vi "Initialize.vi"(7 "writer buffer size":i32=4096, 8 "error in (no error)":errorcluster, 10 "reader url":string, 11 "writer name":string) -> (0 "error out":errorcluster, 3 "NetworkStreamWriter out":refnum<class "NetworkStreamWriter.lvclass">)   [LabVIEW 2011, in "NetworkStreamWriter.lvclass"]
doc: "Instantiates an instance of the NetworkStreamWriter class. A NetworkStreamWriter Object is a wrapper around the LabVIEW Network Stream Writer. The wrapper provides a reconnectable connection and separates writes to the Object from network communication. As with network streams, the writer url on the reader or the reader url on the writer must be given in order to establish the connection. The Object will write data across the network stream at a fixed rate in the background. This allows an application to write data to the Object in time-critical loops, as network communication occurs in a separate loop in the background.\n\n<b>It is critical that all initialized NetworkStreamWriter Objects are closed with the Close method.</b> This method signals the background process to stop. If the Close method is not called, the background process will continue to run on the host computer. For this reason, <b>do not abort an application which uses NetworkStreamWriter Objects.</b>\n\nNote that <b>the NetworkStreamWriter Object is implemented to work by-reference</b>, meaning that copies of an initialized NetworkStreamWriter Object will write to the same network stream internally.\n\nJared Kirschner, 2012."
uses:
  NetworkStreamWriter.lvclass
  Shared/TimeStampedMessage.ctl
  Shared/TimeStampedMessageQueue.ctl
  WriterParameters.ctl
  NetworkStreamWriter.lvclass/NetworkStreamWriter.ctl
  WriterDaemon.vi
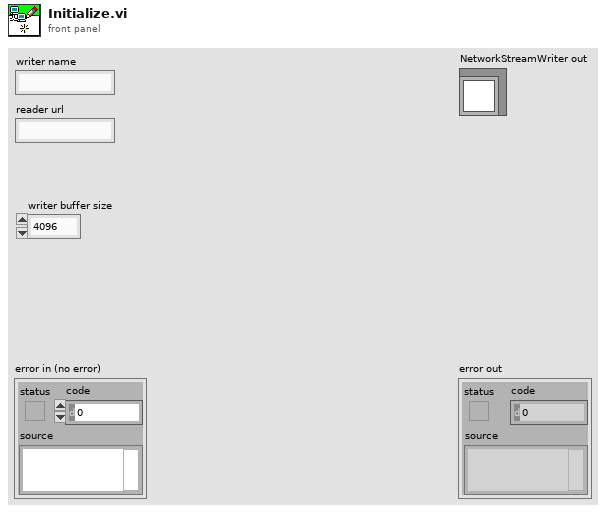
[diagram p1: front panel]
types:
  T1 = typedef "NetworkStreamWriter.lvclass/WriterParameters.ctl" = cluster{"writer name":string, "reader url":string, "writer buffer size":i32}
  T2 = typedef "TimeStampedMessageQueue.ctl" = refnum<queue>
  T3 = typedef "TimeStampedMessage.ctl" = cluster{"Data":variant, "Time Stamp":timestamp}
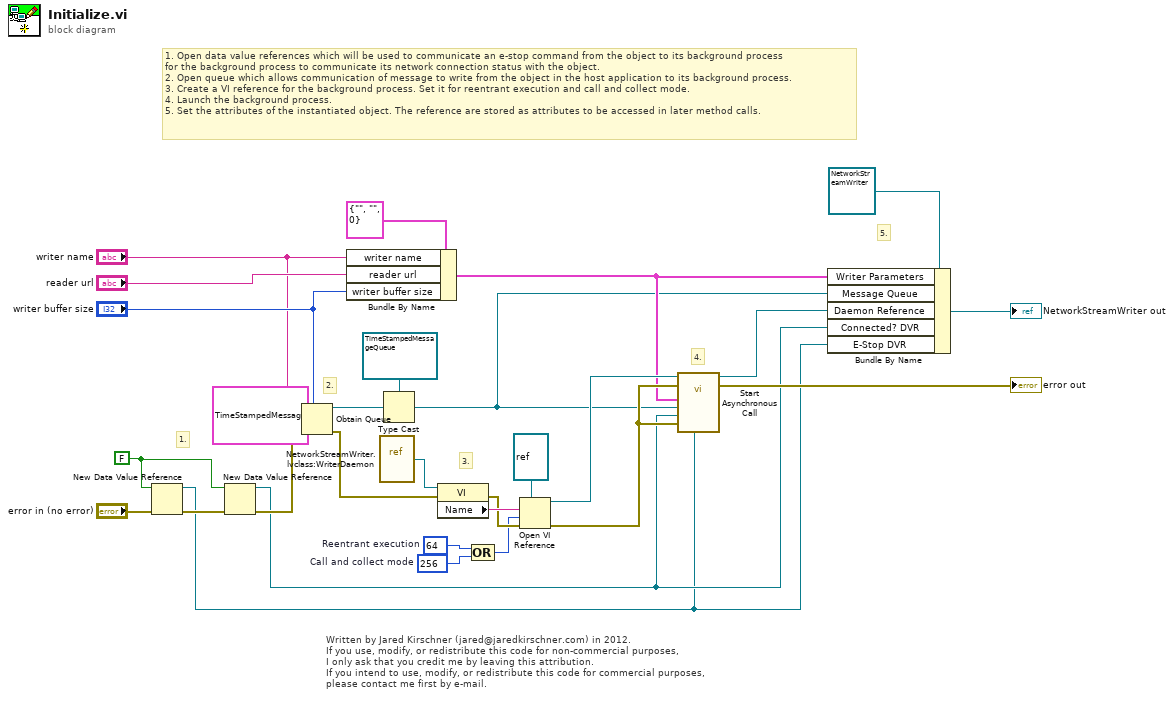
[diagram p0: block diagram]
diagram:
  w10 = FALSE
  w23 = 64  # Reentrant execution
  w24 = 256  # Call and collect mode
  # "1. Open data value references which will be used to communicate an e-stop command from the object to its background process\nfor the background process to communicate its network connection status with the object.\n2. Open queue which allows communication of message to write from the object in the host application to its background process.\n3. Create a VI reference for the background process. Set it for reentrant execution and call and collect mode.\n4. Launch the background process.\n5. Set the attributes of the instantiated object. The reference are stored as attributes to be accessed in later method calls."
  # "5."
  # "4."
  # "3."
  # "2."
  # "1."
  # "Written by Jared Kirschner (jared@jaredkirschner.com) in 2012.\nIf you use, modify, or redistribute this code for non-commercial purposes,\nI only ask that you credit me by leaving this attribution.\nIf you intend to use, modify, or redistribute this code for commercial purposes,\nplease contact me first by e-mail."
  n1 = New Data Value Reference(data value=w10, error in="error in (no error)") -> (data value reference=w5:refnum<data-value>, error out=w7:errorcluster)
  n2 = New Data Value Reference(data value=w10, error in=w7) -> (data value reference=w6:refnum<data-value>, error out=w9:errorcluster)
  n3 = Obtain Queue(max queue size (-1, unlimited)="writer buffer size", name (unnamed)="writer name", element data type=T3 {"Data"=variant, "Time Stamp"=timestamp(0 s since 1904-01-01)}, error in (no error)=w9) -> (queue out=w21:refnum<queue>, error out=w11:errorcluster)  [unwired: 1 in, 1 out]
  n4 = Bundle By Name(cluster=T1 {"writer name"="", "reader url"="", "writer buffer size"=0} ("Writer Parameters"), "writer name"="writer name", "reader url"="reader url", "writer buffer size"="writer buffer size") -> (w2:T1)
  n5 = vi-ref "NetworkStreamWriter.lvclass:WriterDaemon.vi"() -> (w28:refnum<vi>)
  n6 = Type Cast(type=T2 refnum ("Variant Queue"), x=w21) -> (*(type *) &x=w1:T2)
  n7 = property class="VI"(reference=w28, error in=w11) -> (error out=w25:errorcluster, "Name"=w27:string)  [unwired: 1 out]
  n8 = Compound Arithmetic op=OR(w23, w24) -> (w22:i32)
  n9 = Open VI Reference(type specifier VI Refnum (for type only)=refnum<vi> refnum, vi path=w27, options=w22, error in (no error)=w25) -> (vi reference=w19:refnum<vi>, error out=w8:errorcluster)  [unwired: 2 in]
  n10 = call-by-ref "Start Asynchronous Call"(reference=w19, error in=w8, "E-Stop DVR"=w5, 8:"error in (no error)"=w8, "Connected? DVR"=w6, "Message Queue"=w1, "Writer Parameters"=w2) -> (reference out=w4:refnum<vi>, error out=→"error out":errorcluster)  [unwired: 6 in, 1 out]
  n11 = Bundle By Name(cluster=refnum<class "NetworkStreamWriter.lvclass"> refnum ("NetworkStreamWriter out"), "Writer Parameters"=w2, "Message Queue"=w1, "Daemon Reference"=w4, "Connected? DVR"=w6, "E-Stop DVR"=w5) -> (→"NetworkStreamWriter out":refnum<class "NetworkStreamWriter.lvclass">)
